vi "PCO Edge_Cam.vi"(0 "Operation":T2(ring), 1 "Camera-specific in":variant, 5 "Exposure time (s)":dbl, 7 "Save path":path, 9 "Capture mode":enum16{"Single frame", "Sequence"}(ring), 12 "Image in":variant, 14 "Frames in sequence":u32=1 min=1) -> (3 "Camera-specific out":variant, 4 "Status":T1)   [LabVIEW 2015]
uses:
  <vilib>/vision/Image Controls.llb/IMAQ Image.ctl
panel:
  in  "Capture button":refnum<vi>
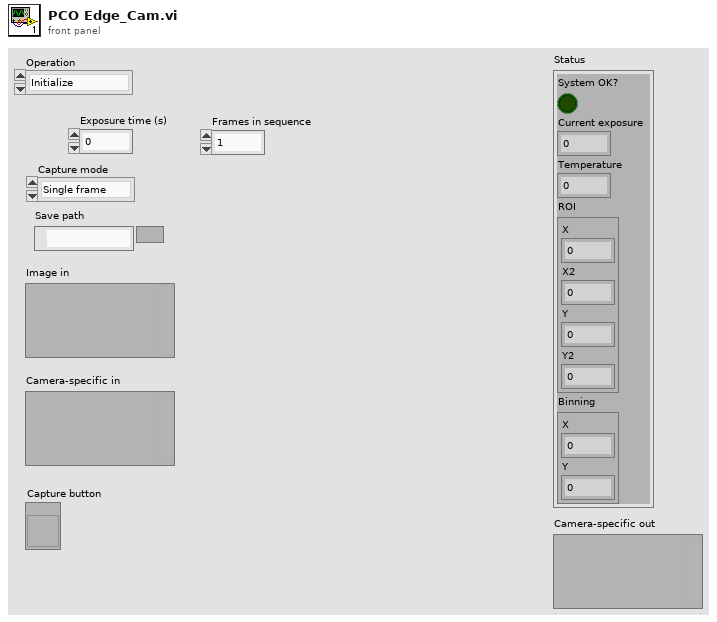
[diagram p1: front panel]
types:
  T1 = cluster{"System OK?":bool, "Current exposure":dbl, "Temperature":dbl, "ROI":cluster{"X":u32, "X2":u32, "Y":u32, "Y2":u32}, "Binning":cluster{"X":u32, "Y":u32}}
  T2 = enum16{"Initialize", "Shut down", "Set capture mode", "Set exposure", "Trigger and read", "Get status", "Other settings"}
  T3 = cluster{"Handle":u64, "Buffers":i16[], "Frames in sequence":u32}
  T4 = cluster{"Size":u16, "InterfaceType":u16, "Camera Number":u16, "CameraNumAtInterface":u16, "OpenFlags":u16[], "OpenDWFlags":u32[], "OpenPtrs":u32[]}
  T5 = typedef "IMAQ Image.ctl" = refnum<image>
  T6 = cluster{"New Image":T5, "Image":refnum<vi>, "FPS target":dbl}
  T7 = enum16{"big-endian, network order", "native, host order", "little-endian"}
  T8 = enum16{"open", "replace", "create", "open or create", "replace or create", "replace or create with confirmation"}
  T9 = cluster{"SSize":u16, "CamType":u16, "CamsSubType":u16, "SerialNumber":u32, "HWVersion":u32, "FWVersion ":u32, "InterfaceType":u16, "HardwareVersions":cluster{"Board":u16, cluster{"string":string, "BatchNumber":u16, "MinorRevision":u8, "MajorRevision":u8, "Variant":u16}[]}, "FirmwareVersions":cluster{"DeviceNum":u16, cluster{"string":string, "MinorRevision":u8, "MajorRevision":u8, "Variant":u16}[]}}
  T10 = cluster{"Size":u16, "SensorTypeDESC":u16, "SensorSubtypeDESC":u16, "MaxHorizontalResStdDESC":u16, "MaxVerticalResStdDESC":u16, "MaxHorizontalResExtDESC":u16, "MaxVerticalResExtDESC":u16, "DynResDESC":u16, "MaxBinHorzDESC":u16, "BinHorzStepDESC":bool, "MaxBinVertDESC":u16, "BinVertStepDESC":bool, "ROIHorzStepDESC":u16, "ROIVertStepDESC":u16, "NumADCDESC":u16, "IRDESC":bool, "MinDelayDESC":u32, "MaxDelayDESC":u32, "MinDelayStepDESC":u32, "MinExpoDESC":u32, "MaxExpoDESC":u32, "MinExpoStepDESC":u32, "MinDelayIRDESC":u32, "MaxDelayIRDESC":u32, "MinExpoIRDESC":u32, "MaxExpoIRDESC":u32, "TimeTableDESC":bool, "DoubleImageDESC":bool, "MinCoolSetDESC":i16, "MaxCoolSetDESC":i16, "MDefaultCoolSetDESC":i16, "PowerDownModeDESC":bool, "OffsetRegDESC":bool, "ColorPattern":cluster{"UpperLeftColor":u8, "UpperRightColor":u8, "LowerLeftColor":u8, "LowerRightColor":u8}, "PatternTypeDESC":bool, "PixelRates":u32[], "CoversionFactors":u16[], "Reserved":u32[], "GeneralCapabilities":u32, "GeneralCapabilities 2":u32, "Min Size Hor":u16, "Min Size Vert":u16, "Ext Synch Freq":u32[], "Cooling Setpoints":i16[], "Soft ROI Hor Step":u16, "Soft ROI Vert Step":u16}
  T11 = cluster{"File refnum":refnum<file>, "Image File Directory":cluster{cluster{"Field":u16, "Type":u16, "Count":u32, "Value / Offset":u32, "Add IFD Offset?":bool}[], cluster{"Data":u32[], "Add offset?":bool}[]}, "Big endian?":bool, "IFD Offset Size":u32}
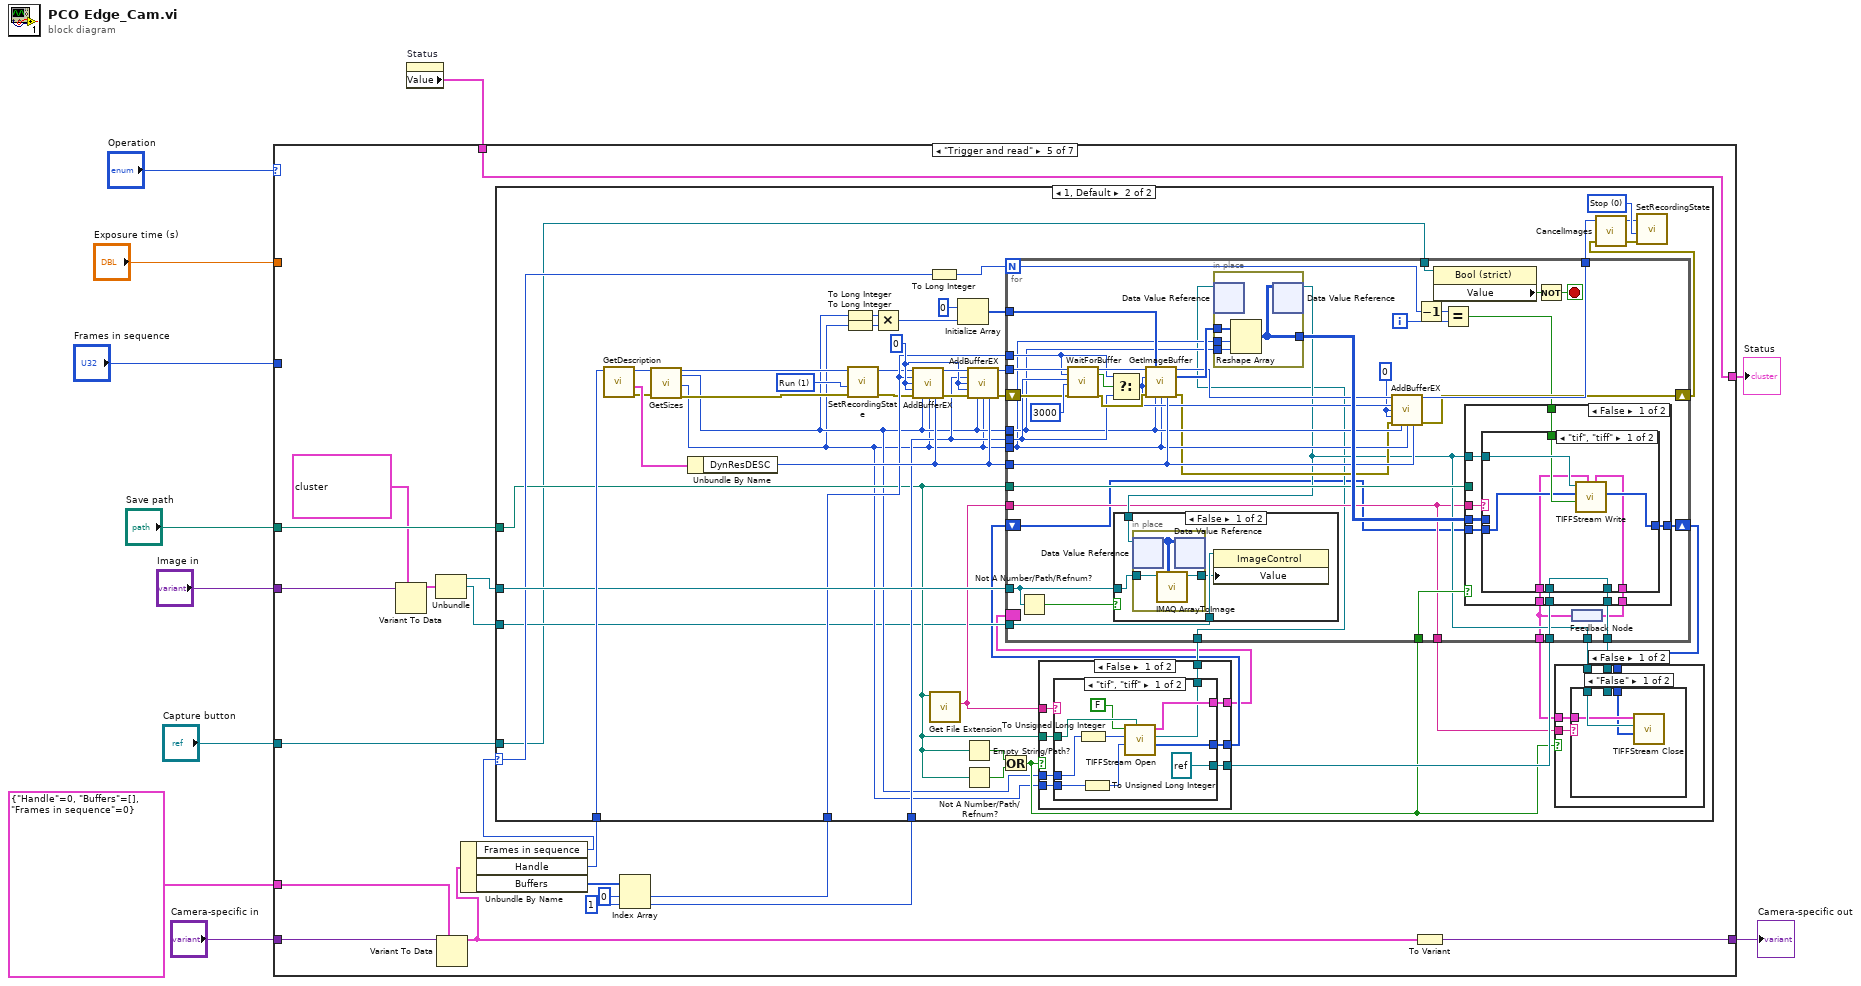
[diagram p0: block diagram]
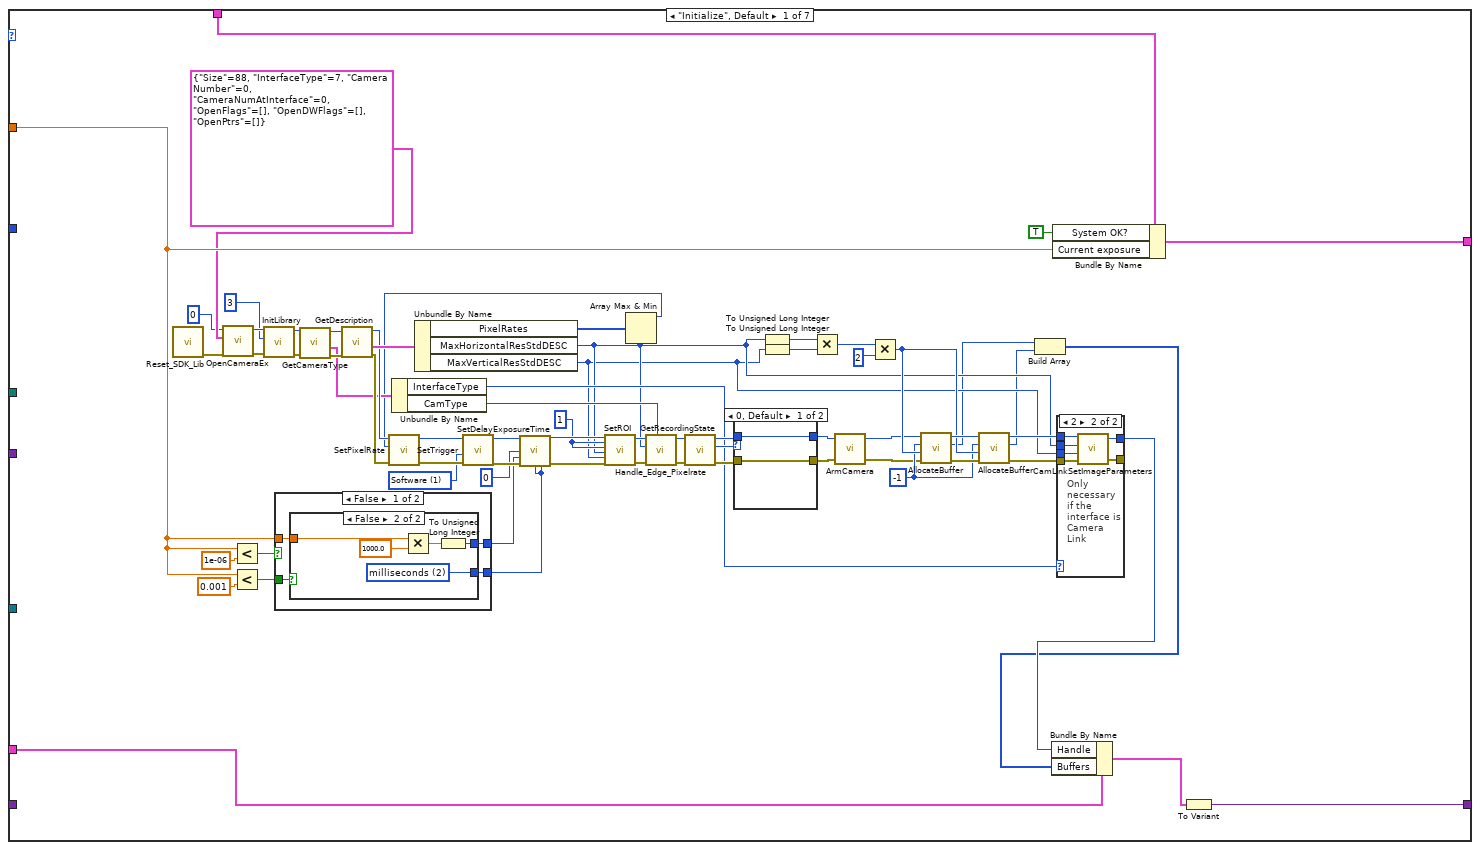
[diagram p2: hidden frame]
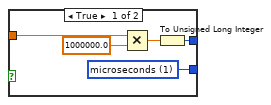
[diagram p3: hidden frame]
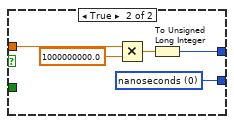
[diagram p4: hidden frame]
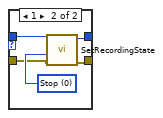
[diagram p6: hidden frame]
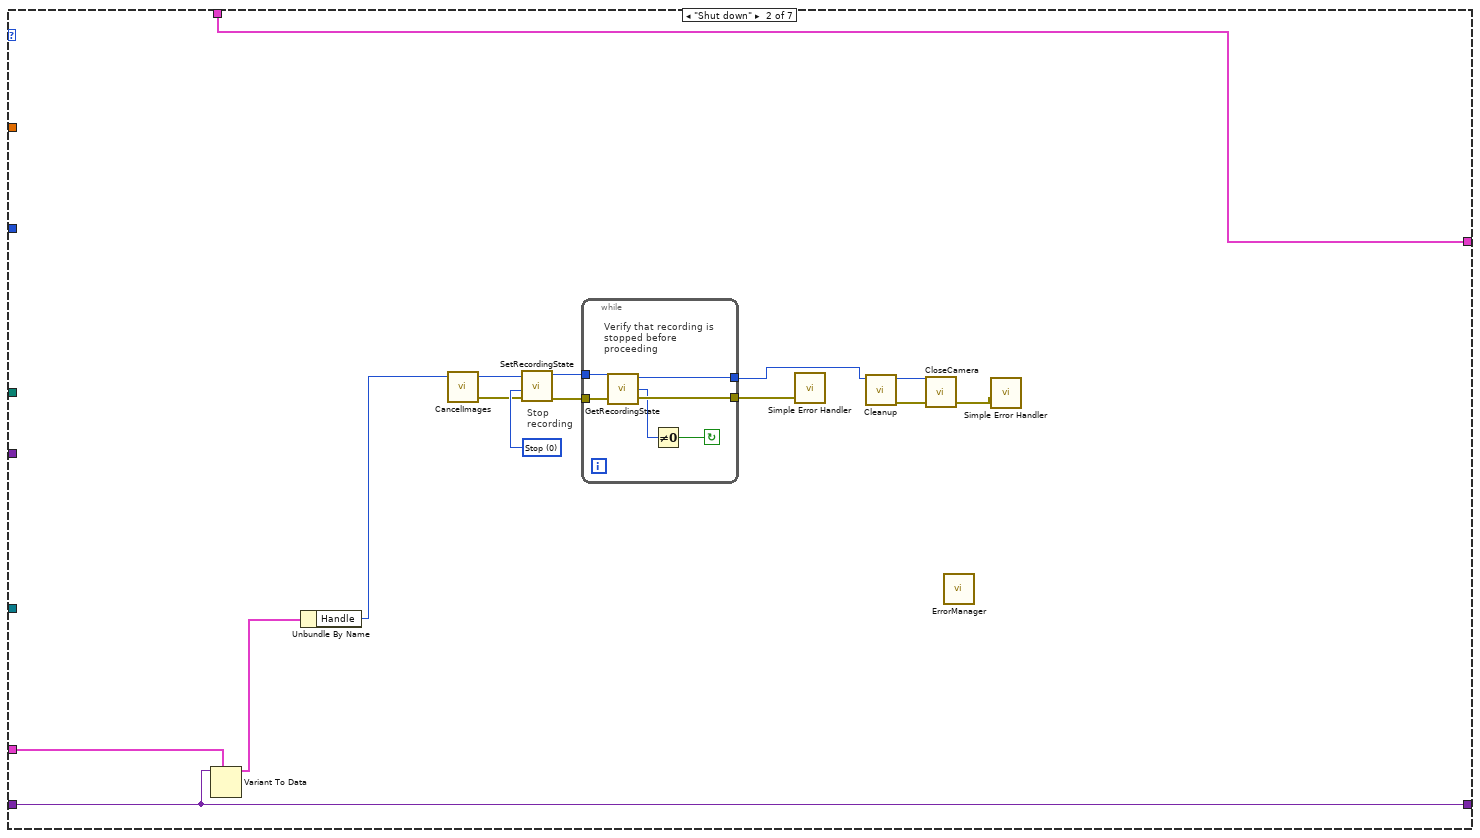
[diagram p7: hidden frame]
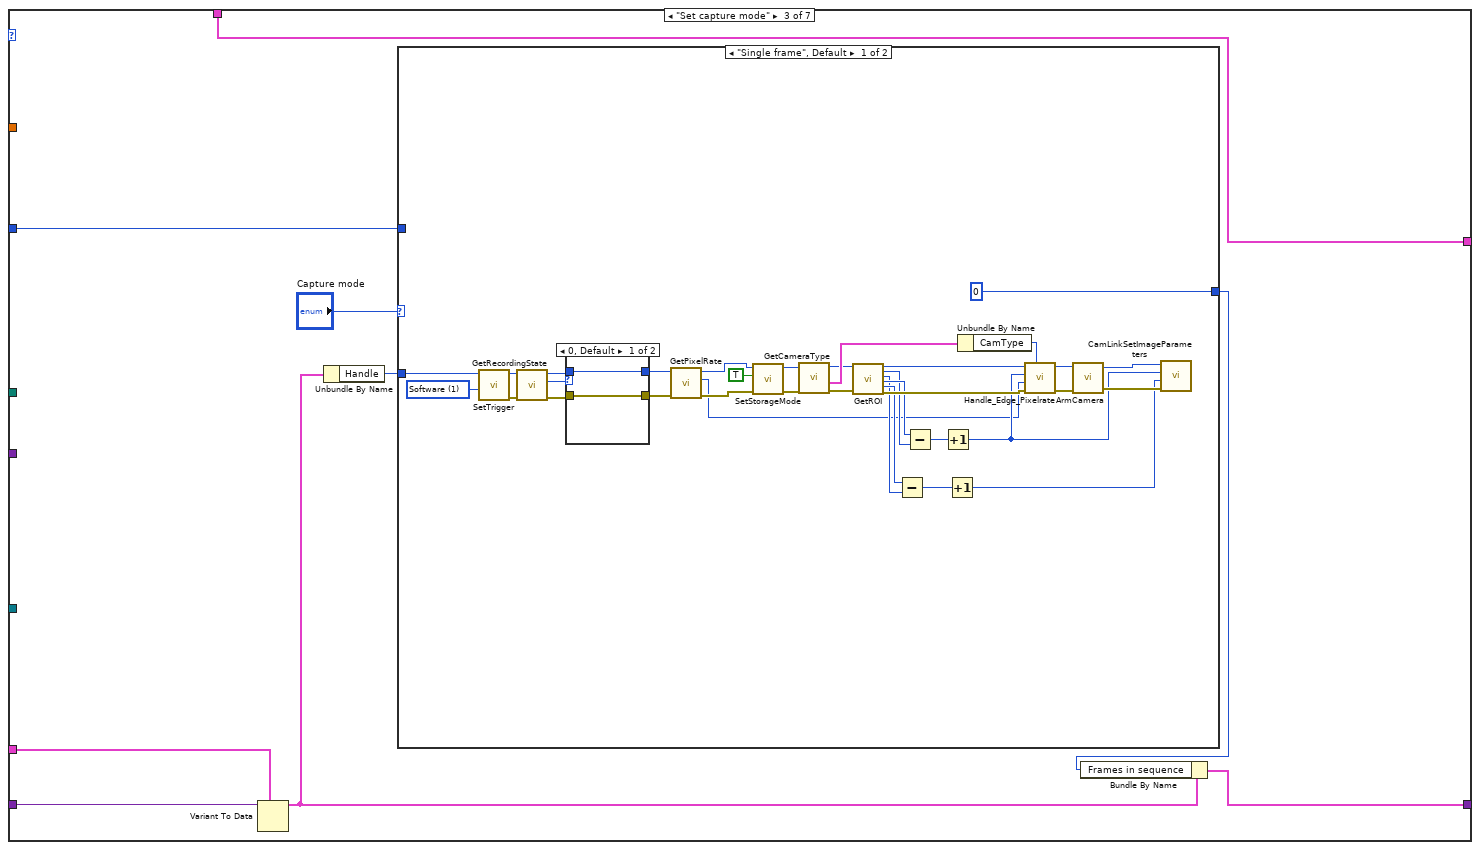
[diagram p8: hidden frame]
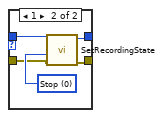
[diagram p9: hidden frame]
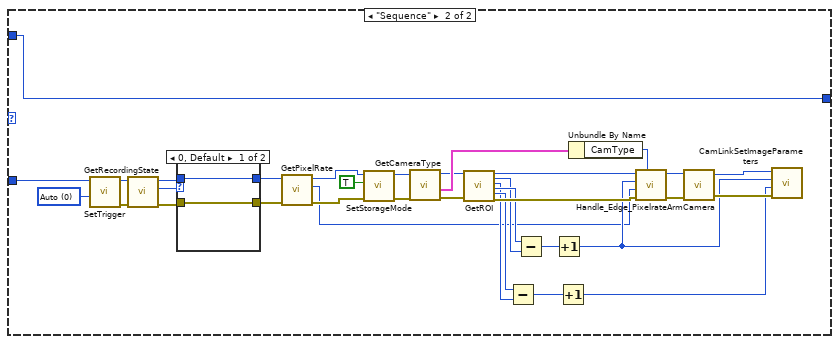
[diagram p10: hidden frame]
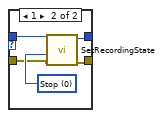
[diagram p11: hidden frame]
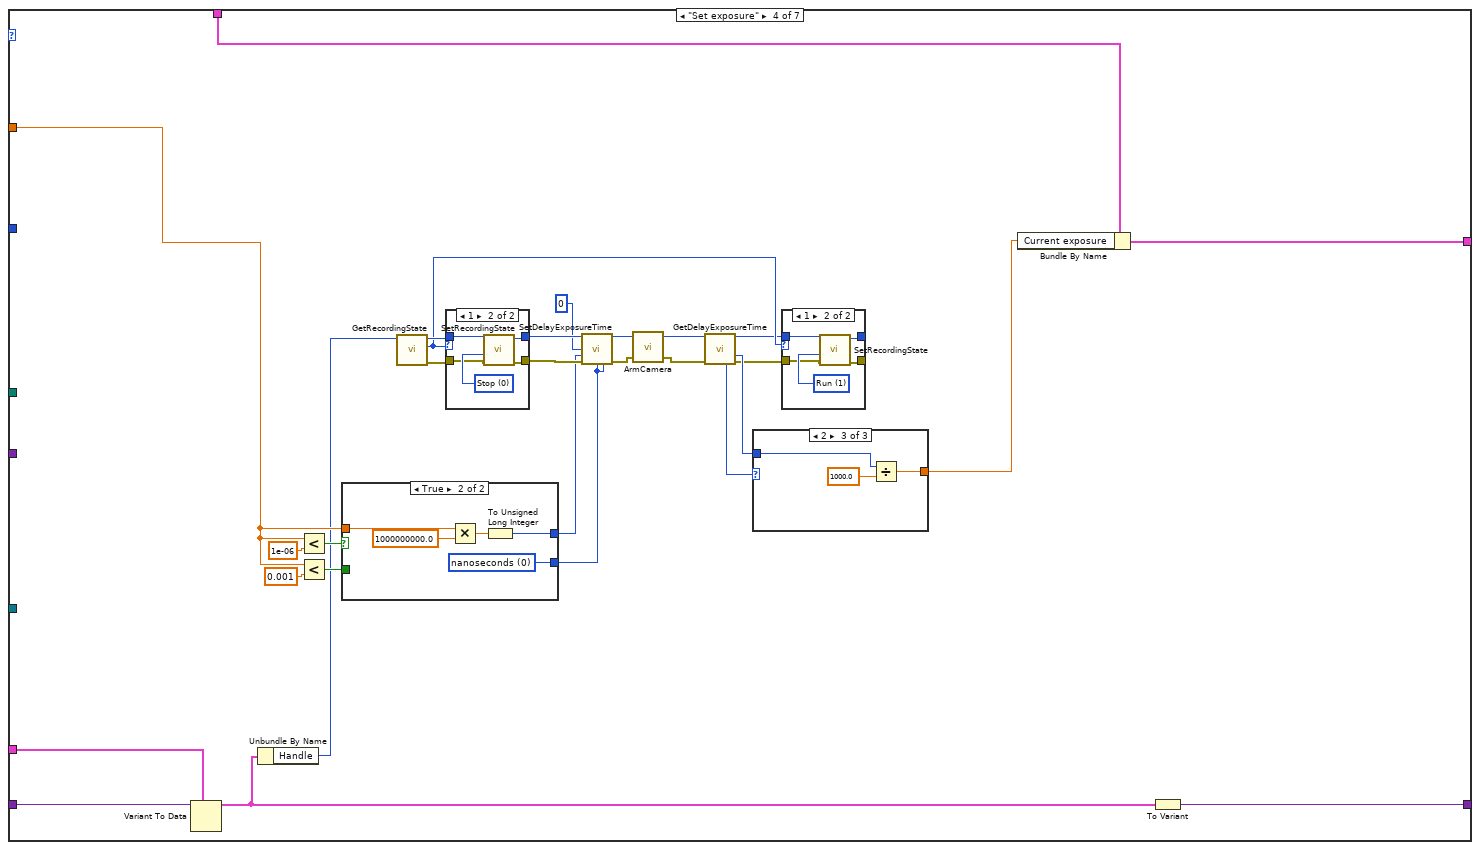
[diagram p12: hidden frame]
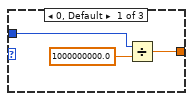
[diagram p14: hidden frame]
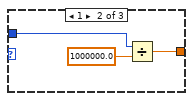
[diagram p15: hidden frame]
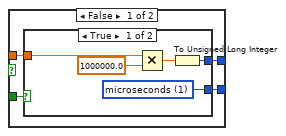
[diagram p16: hidden frame]
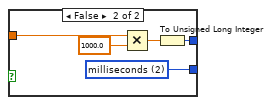
[diagram p17: hidden frame]
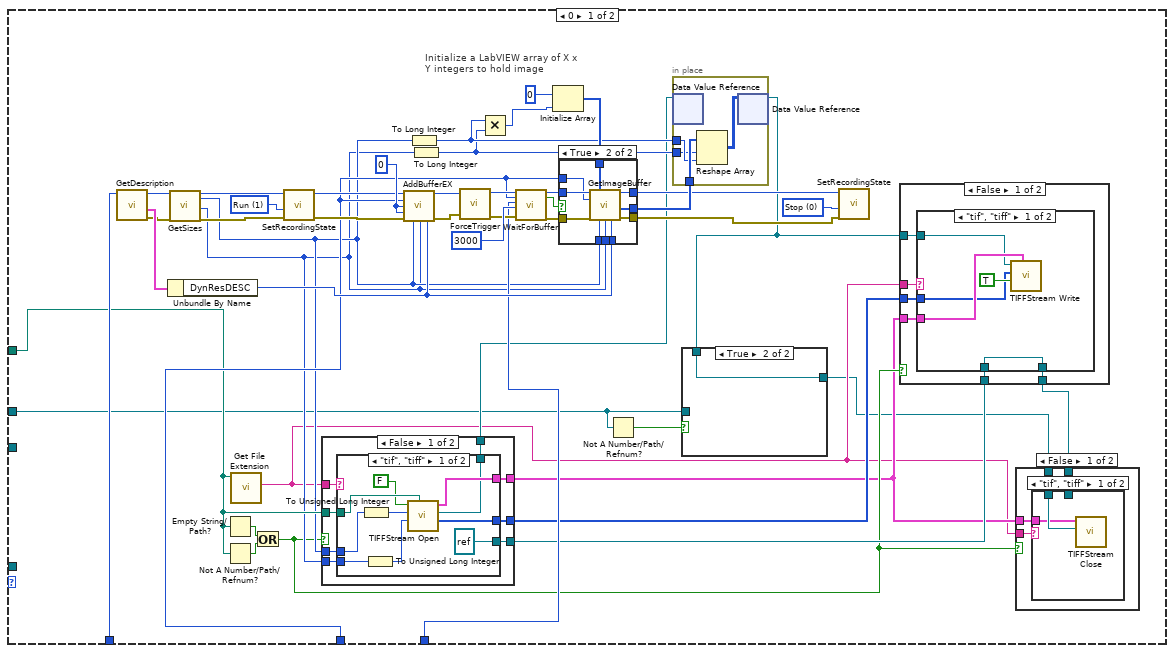
[diagram p19: hidden frame]
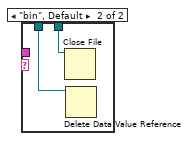
[diagram p20: hidden frame]
diagram:
  n1 = property on="Status" class="Clust (strict)"() -> ("Value"=w9:T1)  [unwired: 2 in, 2 out]
  n2 = case shown="\"Trigger and read\"" "Operation" {
    tunnel: "Exposure time (s)" -> [w27 _ _ w241 _ _ _]
    tunnel: w9 -> [w78 w127 w142 w253 w314 w631 w640]
    tunnel: [w77 w127 w142 w252 w314 w630 w640] -> w8
    tunnel: "Save path" -> [_ _ _ _ w306 _ _]
    tunnel: "Image in" -> [_ _ _ _ w299 _ _]
    tunnel: "Camera-specific in" -> [_ w115 w136 w229 w305 w625 w639]
    tunnel: [w16 w115 w139 w225 w302 w625 w633] -> w3
    tunnel: "Frames in sequence" -> [_ _ w140 _ _ _ _]
    tunnel: T3 {"Handle"=0, "Buffers"=[], "Frames in sequence"=0} -> [w14 w114 w137 w227 w304 _ w635]
    tunnel: "Capture button" -> [_ _ _ _ w296 _ _]
    frame "Initialize", Default {
      w23 = u16 1 ("ROIX0")
      w32 = u16 1 items=["Auto", "Software", "External sequence start ", "External exposure control"] ("TriggerMode")
      w56 = i16 -1
      n3 = call <userlib>:"Reset_SDK_Lib.vi"() -> ("ErrorOut"=w68:errorcluster)  [unwired: 11 in]
      n4 = call <userlib>:"OpenCameraEx.vi"("error in (no error)"=w68, "OpenStructureIn"=T4 {"Size"=88, "InterfaceType"=7, "Camera Number"=0, "CameraNumAtInterface"=0, "OpenFlags"=[], "OpenDWFlags"=[], "OpenPtrs"=[]}, "ph"=u64 0) -> ("error out"=w72:errorcluster, "hout"=w73:u64)  [unwired: 1 in, 2 out]
      n5 = Less?(x=w27, y=1e-06) -> (x < y?=w29:bool)
      n6 = Less?(x=w27, y=0.001) -> (x < y?=w28:bool)
      n7 = call <userlib>:"InitLibrary.vi"("error in (no error)"=w72, "InterfaceType"=u32 3, "ph"=w73) -> ("error out"=w71:errorcluster, "hout"=w70:u64)  [unwired: 7 in]
      n8 = case shown="False" w29 {
        tunnel: [w80 w97] -> w25
        tunnel: w28 -> [w82 _]
        tunnel: w27 -> [w81 w96]
        tunnel: [w79 w93] -> w26
        frame False {
          n9 = case shown="False" w82 {
            tunnel: w81 -> [w84 w89]
            tunnel: [w87 w92] -> w80
            tunnel: [w83 w88] -> w79
            frame True {
              w87 = u16 1 items=["nanoseconds", "microseconds", "milliseconds"] ("ExposureTimeBase")
              n10 = Multiply(x=w84, y=1000000.0) -> (x*y=w85:dbl)
              n11 = To Unsigned Long Integer(number=w85) -> (unsigned 32bit integer=w83:u32)
            }
            frame False {
              w92 = u16 2 items=["nanoseconds", "microseconds", "milliseconds"] ("ExposureTimeBase")
              n12 = Multiply(x=w89, y=1000.0) -> (x*y=w90:dbl)
              n13 = To Unsigned Long Integer(number=w90) -> (unsigned 32bit integer=w88:u32)
            }
          }
        }
        frame True {
          w97 = u16 0 items=["nanoseconds", "microseconds", "milliseconds"] ("ExposureTimeBase")
          n14 = Multiply(x=w96, y=1000000000.0) -> (x*y=w94:dbl)
          n15 = To Unsigned Long Integer(number=w94) -> (unsigned 32bit integer=w93:u32)
        }
      }
      n16 = call <userlib>:"GetCameraType.vi"("ph"=w70, "error in (no error)"=w71) -> ("hout"=w75:u64, "CameraType"=w37:T9, "error out"=w74:errorcluster)  [unwired: 1 in, 1 out]
      n17 = call <userlib>:"GetDescription.vi"("ErrorIn"=w74, "ph"=w75) -> ("ErrorOut"=w47:errorcluster, "Description"=w63:T10, "hout"=w46:u64)  [unwired: 2 in, 1 out]
      n18 = Unbundle By Name(w37) -> ("InterfaceType"=w36:u16, "CamType"=w35:u16)
      n19 = Unbundle By Name(w63) -> ("PixelRates"=w34:u32[], "MaxHorizontalResStdDESC"=w22:u16, "MaxVerticalResStdDESC"=w21:u16)
      n20 = Array Max & Min(array=w34) -> (max value=w33:u32)  [unwired: 3 out]
      n21 = call <userlib>:"SetPixelRate.vi"("error in (no error)"=w47, "PixelRate"=w33, "ph"=w46) -> ("error out"=w54:errorcluster, "hout"=w55:u64)  [unwired: 2 in, 1 out]
      n22 = call <userlib>:"SetTrigger.vi"("error in (no error)"=w54, "TriggerMode"=w32, "ph"=w55) -> ("error out"=w52:errorcluster, "hout"=w53:u64)  [unwired: 2 in, 1 out]
      n23 = call <userlib>:"SetDelayExposureTime.vi"("ph"=w53, "Delay"=u32 0, "Exposure"=w26, "error in (no error)"=w52, "DelayTimeBase"=w25, "ExposureTimeBase"=w25) -> ("hout"=w49:u64, "error out"=w51:errorcluster)  [unwired: 7 in, 1 out]
      n24 = call <userlib>:"SetROI.vi"("ph"=w49, "ROIX0"=w23, "ROIY0"=w23, "ROIX1"=w22, "ROIY1"=w21, "error in (no error)"=w51) -> ("hout"=w48:u64, "error out"=w50:errorcluster)  [unwired: 12 in]
      n25 = call <userlib>:"Handle_Edge_Pixelrate.vi"("Cameratype"=w35, "error in (no error)"=w50, "X-Resolution"=w22, "ph"=w48) -> ("error out"=w44:errorcluster, "hout"=w45:u64)  [unwired: 6 in]
      n26 = call <userlib>:"GetRecordingState.vi"("ErrorIn"=w44, "ph"=w45) -> ("ErrorOut"=w60:errorcluster, "Error"=w58:i32, "hout"=w61:u64)  [unwired: 2 in, 1 out]
      n27 = case shown="0, Default" w58 {
        tunnel: w61 -> [w107 w111]
        tunnel: w60 -> [w106 w110]
        tunnel: [w107 w109] -> w43
        tunnel: [w106 w108] -> w41
        frame 0, Default {
        }
        frame 1 {
          w112 = u16 0 items=["Stop", "Run"] ("RecordingState")
          n28 = call <userlib>:"SetRecordingState.vi"("ErrorIn"=w110, "RecordingState"=w112, "ph"=w111) -> ("ErrorOut"=w108:errorcluster, "hout"=w109:u64)  [unwired: 2 in, 1 out]
        }
      }
      n29 = To Unsigned Long Integer(number=w22) -> (unsigned 32bit integer=w65:u32)
      n30 = To Unsigned Long Integer(number=w21) -> (unsigned 32bit integer=w64:u32)
      n31 = Multiply(x=w65, y=w64) -> (x*y=w66:u32)
      n32 = call <userlib>:"ArmCamera.vi"("error in (no error)"=w41, "ph"=w43) -> ("error out"=w40:errorcluster, "hout"=w42:u64)  [unwired: 1 in, 1 out]
      n33 = Multiply(x=w66, y=u32 2) -> (x*y=w57:u32)
      n34 = call <userlib>:"AllocateBuffer.vi"("error in (no error)"=w40, "Size"=w57, "BufNr"=w56, "ph"=w42) -> ("error out"=w62:errorcluster, "BufNrOut"=w20:i16, "hout"=w59:u64)  [unwired: 2 in, 3 out]
      n35 = call <userlib>:"AllocateBuffer.vi"("error in (no error)"=w62, "Size"=w57, "BufNr"=w56, "ph"=w59) -> ("error out"=w38:errorcluster, "BufNrOut"=w19:i16, "hout"=w39:u64)  [unwired: 2 in, 3 out]
      n36 = Build Array(w20, w19) -> (w17:i16[])
      n37 = Bundle By Name(cluster=w78, "System OK?"=TRUE, "Current exposure"=w27) -> (w77:T1)
      n38 = case shown="2" w36 {
        tunnel: w38 -> [w98 w105]
        tunnel: [w98 w104] -> _
        tunnel: w39 -> [w99 w103]
        tunnel: [w99 w102] -> w18
        tunnel: w21 -> [_ w101]
        tunnel: w22 -> [_ w100]
        frame 0, Default {
        }
        frame 2 {
          # "Only necessary if the interface is Camera Link"
          n39 = call <userlib>:"CamLinkSetImageParameters.vi"("error in (no error)"=w105, "YRes"=w101, "XRes"=w100, "ph"=w103) -> ("error out"=w104:errorcluster, "hout"=w102:u64)  [unwired: 1 out]
        }
      }
      n40 = Bundle By Name(cluster=w14, "Handle"=w18, "Buffers"=w17) -> (w15:T3)
      n41 = To Variant(anything=w15) -> (Variant=w16:variant)
    }
    frame "Shut down" {
      w126 = u16 0 items=["Stop", "Run"] ("RecordingState")
      # "Stop recording"
      n42 = Variant To Data(type=w114, Variant=w115) -> (data=w113:T3)  [unwired: 1 in, 1 out]
      n43 = Unbundle By Name(w113) -> ("Handle"=w116:u64)
      n44 = call <userlib>:"CancelImages.vi"("ph"=w116) -> ("error out"=w123:errorcluster, "hout"=w122:u64)  [unwired: 2 in, 1 out]
      n45 = call <userlib>:"SetRecordingState.vi"("ErrorIn"=w123, "RecordingState"=w126, "ph"=w122) -> ("ErrorOut"=w124:errorcluster, "hout"=w125:u64)  [unwired: 2 in, 1 out]
      n46 = while {
        tunnel: [w131] -> w121
        tunnel: w124 -> [w132]
        tunnel: w125 -> [w133]
        tunnel: [w128] -> w117
        stop <- w129 continue-if-true
        # "Verify that recording is stopped before proceeding"
        n47 = call <userlib>:"GetRecordingState.vi"("ErrorIn"=w132, "ph"=w133) -> ("ErrorOut"=w131:errorcluster, "RecordingState"=w130:u16, "hout"=w128:u64)  [unwired: 2 in, 1 out]
        n48 = Not Equal To 0?(x=w130) -> (x != 0?=w129:bool)
      }
      n49 = call <vilib>:"Simple Error Handler.vi"("error in (no error)"=w121) -> ()  [unwired: 4 in, 5 out]
      n50 = call <userlib>:"Cleanup.vi"("ph"=w117) -> ("error out"=w118:errorcluster, "hout"=w119:u64)  [unwired: 9 in]
      n51 = call <userlib>:"CloseCamera.vi"("ErrorIn"=w118, "Handle in"=w119) -> ("ErrorOut"=w120:errorcluster)  [unwired: 1 in, 2 out]
      n52 = call <userlib>:"ErrorManager.vi"() -> ()  [unwired: 5 in, 1 out]
      n53 = call <vilib>:"Simple Error Handler.vi"("error in (no error)"=w120) -> ()  [unwired: 4 in, 5 out]
    }
    frame "Set capture mode" {
      n54 = Variant To Data(type=w137, Variant=w136) -> (data=w135:T3)  [unwired: 1 in, 1 out]
      n55 = Unbundle By Name(w135) -> ("Handle"=w138:u64)
      n56 = case shown="\"Single frame\", Default" "Capture mode" {
        tunnel: w140 -> [_ w184]
        tunnel: [u32 0 ("Frames in sequence") w184] -> w134
        tunnel: w138 -> [w174 w216]
        frame "Single frame", Default {
          w175 = u16 1 items=["Auto", "Software", "External sequence start ", "External exposure control"] ("TriggerMode")
          n57 = call <userlib>:"SetTrigger.vi"("TriggerMode"=w175, "ph"=w174) -> ("error out"=w169:errorcluster, "hout"=w170:u64)  [unwired: 3 in, 1 out]
          n58 = call <userlib>:"GetRecordingState.vi"("ErrorIn"=w169, "ph"=w170) -> ("ErrorOut"=w172:errorcluster, "Error"=w171:i32, "hout"=w173:u64)  [unwired: 2 in, 1 out]
          n59 = case shown="0, Default" w171 {
            tunnel: w173 -> [w178 w182]
            tunnel: w172 -> [w177 w181]
            tunnel: [w178 w180] -> w146
            tunnel: [w177 w179] -> w145
            frame 0, Default {
            }
            frame 1 {
              w183 = u16 0 items=["Stop", "Run"] ("RecordingState")
              n60 = call <userlib>:"SetRecordingState.vi"("ErrorIn"=w181, "RecordingState"=w183, "ph"=w182) -> ("ErrorOut"=w179:errorcluster, "hout"=w180:u64)  [unwired: 2 in, 1 out]
            }
          }
          n61 = call <userlib>:"GetPixelRate.vi"("error in (no error)"=w145, "ph"=w146) -> ("error out"=w144:errorcluster, "PixelRate"=w143:u32, "hout"=w147:u64)  [unwired: 2 in, 1 out]
          n62 = call <userlib>:"SetStorageMode.vi"("error in (no error)"=w144, "StorageMode"=TRUE, "ph"=w147) -> ("error out"=w161:errorcluster, "hout"=w162:u64)  [unwired: 2 in, 1 out]
          n63 = call <userlib>:"GetCameraType.vi"("ph"=w162, "error in (no error)"=w161) -> ("hout"=w157:u64, "CameraType"=w168:T9, "error out"=w159:errorcluster)  [unwired: 1 in, 1 out]
          n64 = call <userlib>:"GetROI.vi"("ph"=w157, "error in (no error)"=w159) -> ("hout"=w156:u64, "ROIX0"=w154:u16, "ROIY0"=w152:u16, "ROIX1"=w155:u16, "ROIY1"=w153:u16, "error out"=w158:errorcluster)  [unwired: 12 in]
          n65 = Subtract(x=w153, y=w152) -> (x-y=w150:u16)
          n66 = Subtract(x=w155, y=w154) -> (x-y=w151:u16)
          n67 = Increment(x=w151) -> (x+1=w149:u16)
          n68 = Increment(x=w150) -> (x+1=w148:u16)
          n69 = Unbundle By Name(w168) -> ("CamType"=w167:u16)
          n70 = call <userlib>:"Handle_Edge_Pixelrate.vi"("Cameratype"=w167, "error in (no error)"=w158, "PixelRate"=w143, "X-Resolution"=w149, "ph"=w156) -> ("error out"=w163:errorcluster, "hout"=w164:u64)  [unwired: 5 in]
          n71 = call <userlib>:"ArmCamera.vi"("error in (no error)"=w163, "ph"=w164) -> ("error out"=w166:errorcluster, "hout"=w165:u64)  [unwired: 1 in, 1 out]
          n72 = call <userlib>:"CamLinkSetImageParameters.vi"("error in (no error)"=w166, "YRes"=w148, "XRes"=w149, "ph"=w165) -> ()  [unwired: 3 out]
        }
        frame "Sequence" {
          w217 = u16 0 items=["Auto", "Software", "External sequence start ", "External exposure control"] ("TriggerMode")
          n73 = call <userlib>:"SetTrigger.vi"("TriggerMode"=w217, "ph"=w216) -> ("error out"=w211:errorcluster, "hout"=w212:u64)  [unwired: 3 in, 1 out]
          n74 = call <userlib>:"GetRecordingState.vi"("ErrorIn"=w211, "ph"=w212) -> ("ErrorOut"=w214:errorcluster, "Error"=w213:i32, "hout"=w215:u64)  [unwired: 2 in, 1 out]
          n75 = case shown="0, Default" w213 {
            tunnel: w215 -> [w219 w223]
            tunnel: w214 -> [w218 w222]
            tunnel: [w219 w221] -> w188
            tunnel: [w218 w220] -> w187
            frame 0, Default {
            }
            frame 1 {
              w224 = u16 0 items=["Stop", "Run"] ("RecordingState")
              n76 = call <userlib>:"SetRecordingState.vi"("ErrorIn"=w222, "RecordingState"=w224, "ph"=w223) -> ("ErrorOut"=w220:errorcluster, "hout"=w221:u64)  [unwired: 2 in, 1 out]
            }
          }
          n77 = call <userlib>:"GetPixelRate.vi"("error in (no error)"=w187, "ph"=w188) -> ("error out"=w186:errorcluster, "PixelRate"=w185:u32, "hout"=w189:u64)  [unwired: 2 in, 1 out]
          n78 = call <userlib>:"SetStorageMode.vi"("error in (no error)"=w186, "StorageMode"=TRUE, "ph"=w189) -> ("error out"=w203:errorcluster, "hout"=w204:u64)  [unwired: 2 in, 1 out]
          n79 = call <userlib>:"GetCameraType.vi"("ph"=w204, "error in (no error)"=w203) -> ("hout"=w199:u64, "CameraType"=w210:T9, "error out"=w201:errorcluster)  [unwired: 1 in, 1 out]
          n80 = call <userlib>:"GetROI.vi"("ph"=w199, "error in (no error)"=w201) -> ("hout"=w198:u64, "ROIX0"=w196:u16, "ROIY0"=w194:u16, "ROIX1"=w197:u16, "ROIY1"=w195:u16, "error out"=w200:errorcluster)  [unwired: 12 in]
          n81 = Subtract(x=w195, y=w194) -> (x-y=w192:u16)
          n82 = Subtract(x=w197, y=w196) -> (x-y=w193:u16)
          n83 = Increment(x=w193) -> (x+1=w191:u16)
          n84 = Increment(x=w192) -> (x+1=w190:u16)
          n85 = Unbundle By Name(w210) -> ("CamType"=w209:u16)
          n86 = call <userlib>:"Handle_Edge_Pixelrate.vi"("Cameratype"=w209, "error in (no error)"=w200, "PixelRate"=w185, "X-Resolution"=w191, "ph"=w198) -> ("error out"=w205:errorcluster, "hout"=w206:u64)  [unwired: 5 in]
          n87 = call <userlib>:"ArmCamera.vi"("error in (no error)"=w205, "ph"=w206) -> ("error out"=w208:errorcluster, "hout"=w207:u64)  [unwired: 1 in, 1 out]
          n88 = call <userlib>:"CamLinkSetImageParameters.vi"("error in (no error)"=w208, "YRes"=w190, "XRes"=w191, "ph"=w207) -> ()  [unwired: 3 out]
        }
      }
      n89 = Bundle By Name(cluster=w135, "Frames in sequence"=w134) -> (w139:T3)
    }
    frame "Set exposure" {
      n90 = Variant To Data(type=w227, Variant=w229) -> (data=w226:T3)  [unwired: 1 in, 1 out]
      n91 = Unbundle By Name(w226) -> ("Handle"=w228:u64)
      n92 = Less?(x=w241, y=1e-06) -> (x < y?=w243:bool)
      n93 = Less?(x=w241, y=0.001) -> (x < y?=w242:bool)
      n94 = case shown="True" w243 {
        tunnel: [w271 w288] -> w238
        tunnel: w242 -> [w273 _]
        tunnel: w241 -> [w272 w287]
        tunnel: [w270 w284] -> w239
        frame False {
          n95 = case shown="True" w273 {
            tunnel: w272 -> [w275 w280]
            tunnel: [w278 w283] -> w271
            tunnel: [w274 w279] -> w270
            frame True {
              w278 = u16 1 items=["nanoseconds", "microseconds", "milliseconds"] ("ExposureTimeBase")
              n96 = Multiply(x=w275, y=1000000.0) -> (x*y=w276:dbl)
              n97 = To Unsigned Long Integer(number=w276) -> (unsigned 32bit integer=w274:u32)
            }
            frame False {
              w283 = u16 2 items=["nanoseconds", "microseconds", "milliseconds"] ("ExposureTimeBase")
              n98 = Multiply(x=w280, y=1000.0) -> (x*y=w281:dbl)
              n99 = To Unsigned Long Integer(number=w281) -> (unsigned 32bit integer=w279:u32)
            }
          }
        }
        frame True {
          w288 = u16 0 items=["nanoseconds", "microseconds", "milliseconds"] ("ExposureTimeBase")
          n100 = Multiply(x=w287, y=1000000000.0) -> (x*y=w285:dbl)
          n101 = To Unsigned Long Integer(number=w285) -> (unsigned 32bit integer=w284:u32)
        }
      }
      n102 = call <userlib>:"GetRecordingState.vi"("ph"=w228) -> ("ErrorOut"=w250:errorcluster, "Error"=w233:i32, "hout"=w251:u64)  [unwired: 3 in, 1 out]
      n103 = case shown="1" w233 {
        tunnel: w251 -> [w290 w294]
        tunnel: w250 -> [w289 w293]
        tunnel: [w290 w292] -> w249
        tunnel: [w289 w291] -> w246
        frame 0, Default {
        }
        frame 1 {
          w295 = u16 0 items=["Stop", "Run"] ("RecordingState")
          n104 = call <userlib>:"SetRecordingState.vi"("ErrorIn"=w293, "RecordingState"=w295, "ph"=w294) -> ("ErrorOut"=w291:errorcluster, "hout"=w292:u64)  [unwired: 2 in, 1 out]
        }
      }
      n105 = call <userlib>:"SetDelayExposureTime.vi"("ph"=w249, "Delay"=u32 0, "Exposure"=w239, "error in (no error)"=w246, "DelayTimeBase"=w238, "ExposureTimeBase"=w238) -> ("hout"=w248:u64, "error out"=w247:errorcluster)  [unwired: 7 in, 1 out]
      n106 = call <userlib>:"ArmCamera.vi"("error in (no error)"=w247, "ph"=w248) -> ("error out"=w236:errorcluster, "hout"=w237:u64)  [unwired: 1 in, 1 out]
      n107 = call <userlib>:"GetDelayExposureTime.vi"("ph"=w237, "error in (no error)"=w236) -> ("hout"=w232:u64, "Exposure"=w234:u32, "ExposureTimeBase"=w235:u16, "error out"=w231:errorcluster)  [unwired: 7 in, 3 out]
      n108 = case shown="2" w235 {
        tunnel: w234 -> [w263 w266 w269]
        tunnel: [w261 w264 w267] -> w230
        frame 0, Default {
          n109 = Divide(x=w263, y=1000000000.0) -> (x/y=w261:dbl)
        }
        frame 1 {
          n110 = Divide(x=w266, y=1000000.0) -> (x/y=w264:dbl)
        }
        frame 2 {
          n111 = Divide(x=w269, y=1000.0) -> (x/y=w267:dbl)
        }
      }
      n112 = case shown="1" w233 {
        tunnel: w232 -> [w255 w259]
        tunnel: w231 -> [w254 w258]
        tunnel: [w255 w257] -> _
        tunnel: [w254 w256] -> _
        frame 0, Default {
        }
        frame 1 {
          w260 = u16 1 items=["Stop", "Run"] ("RecordingState")
          n113 = call <userlib>:"SetRecordingState.vi"("ErrorIn"=w258, "RecordingState"=w260, "ph"=w259) -> ("ErrorOut"=w256:errorcluster, "hout"=w257:u64)  [unwired: 2 in, 1 out]
        }
      }
      n114 = Bundle By Name(cluster=w253, "Current exposure"=w230) -> (w252:T1)
      n115 = To Variant(anything=w226) -> (Variant=w225:variant)
    }
    frame "Trigger and read" {
      n116 = Variant To Data(type=T6 {"New Image"=refnum, "Image"=refnum, "FPS target"=0.0} ("output cluster"), Variant=w299) -> (data=w301:T6)  [unwired: 1 in, 1 out]
      n117 = Unbundle(w301) -> ("New Image"=w298:T5, "Image"=w297:refnum<vi>)  [unwired: 1 out]
      n118 = Variant To Data(type=w304, Variant=w305) -> (data=w303:T3)  [unwired: 1 in, 1 out]
      n119 = Unbundle By Name(w303) -> ("Frames in sequence"=w307:u32, "Handle"=w308:u64, "Buffers"=w313:i16[])
      n120 = Index Array(array=w313, index #1=0 ("index"), index #2=1 ("index")) -> (element #1=w310:i16, element #2=w309:i16)
      n121 = case shown="1, Default" w307 {
        selector: w307 -> [_ w491]
        tunnel: w310 -> [w330 w483]
        tunnel: w309 -> [w329 w485]
        tunnel: w308 -> [w349 w495]
        tunnel: w298 -> [w324 w493]
        tunnel: w306 -> [w328 w462]
        tunnel: w297 -> [_ w454]
        tunnel: w296 -> [_ w451]
        frame 0 {
          w343 = u16 0 items=["Stop", "Run"] ("RecordingState")
          w346 = u16 1 items=["Stop", "Run"] ("RecordingState")
          w356 = u32 0
          # "Initialize a LabVIEW array of X x Y integers to hold image"
          n122 = call <userlib>:"GetDescription.vi"("ph"=w349) -> ("ErrorOut"=w336:errorcluster, "Description"=w348:T10, "hout"=w334:u64)  [unwired: 3 in, 1 out]
          n123 = Unbundle By Name(w348) -> ("DynResDESC"=w347:u16)
          n124 = call <userlib>:"GetSizes.vi"("ph"=w334, "ErrorIn"=w336) -> ("hout"=w333:u64, "XResAct"=w327:u16, "YResAct"=w326:u16, "ErrorOut"=w335:errorcluster)  [unwired: 11 in, 3 out]
          n125 = Empty String/Path?(string/path=w328) -> (empty?=w331:bool)
          n126 = Not A Number/Path/Refnum?(number/path/refnum=w328) -> (NaN/Path/Refnum?=w332:bool)
          n127 = call <vilib>:"Get File Extension.vi"("file"=w328) -> ("lowercase file extension"=w317:string)  [unwired: 6 in, 4 out]
          n128 = Or(x=w331, y=w332) -> (x .or. y?=w320:bool)
          n129 = call <userlib>:"SetRecordingState.vi"("ErrorIn"=w335, "RecordingState"=w346, "ph"=w333) -> ("ErrorOut"=w344:errorcluster, "hout"=w345:u64)  [unwired: 2 in, 1 out]
          n130 = case shown="False" w320 {
            tunnel: w328 -> [w403 _]
            tunnel: [w402 refnum<file> refnum ("refnum out")] -> w323
            tunnel: w317 -> [w401 _]
            tunnel: [w400 _] -> w318
            tunnel: [w399 w426] -> w325
            tunnel: [w398 _] -> w322
            tunnel: w327 -> [w397 w429]
            tunnel: w326 -> [w396 w430]
            frame False {
              n131 = case shown="\"tif\", \"tiff\"" w401 {
                tunnel: w403 -> [w412 w423]
                tunnel: [refnum<file> refnum ("refnum out") w421] -> w402
                tunnel: [w411 _] -> w400
                tunnel: [w410 w416] -> w399
                tunnel: [w409 _] -> w398
                tunnel: w397 -> [w408 w414]
                tunnel: w396 -> [w407 w415]
                frame "tif", "tiff" {
                  n132 = To Unsigned Long Integer(number=w408) -> (unsigned 32bit integer=w405:u32)
                  n133 = To Unsigned Long Integer(number=w407) -> (unsigned 32bit integer=w406:u32)
                  n134 = call "TIFFStream Open.vi"("File path"=w412, "Height Pixels"=w406, "Width Pixels"=w405, "Big endian?"=FALSE) -> ("Current and next IFD offset"=w409:u32[], "Image data reference"=w410:refnum<data-value>, "File data"=w411:T11)  [unwired: 4 in, 1 out]
                }
                frame "bin", Default {
                  n135 = To Long Integer(number=w415) -> (32bit integer=w417:i32)
                  n136 = To Long Integer(number=w414) -> (32bit integer=w418:i32)
                  n137 = Open/Create/Replace File(file path (use dialog)=w423, operation (0:open)=T8."replace or create") -> (refnum out=w421:refnum<file>)  [unwired: 4 in, 2 out]
                  n138 = Initialize Array(u16 0 ("element"), w417, w418) -> (w419:u16[][])
                  n139 = New Data Value Reference(data value=w419) -> (data value reference=w416:refnum<data-value>)  [unwired: 1 in, 1 out]
                }
              }
            }
            frame True {
              n140 = To Long Integer(number=w430) -> (32bit integer=w424:i32)
              n141 = To Long Integer(number=w429) -> (32bit integer=w425:i32)
              n142 = Initialize Array(u16 0 ("element"), w424, w425) -> (w427:u16[][])
              n143 = New Data Value Reference(data value=w427) -> (data value reference=w426:refnum<data-value>)  [unwired: 1 in, 1 out]
            }
          }
          n144 = call <userlib>:"AddBufferEX.vi"("ph"=w345, "BuffNr"=w330, "1stImage"=w356, "LastImage"=w356, "error in (no error)"=w344, "XRes"=w327, "YRes"=w326, "BitPerPixel"=w347) -> ("hout"=w355:u64, "error out"=w354:errorcluster)  [unwired: 5 in, 1 out]
          n145 = To Long Integer(number=w327) -> (32bit integer=w339:i32)
          n146 = To Long Integer(number=w326) -> (32bit integer=w338:i32)
          n147 = call <userlib>:"ForceTrigger.vi"("ph"=w355, "error in (no error)"=w354) -> ("hout"=w352:u64, "error out"=w353:errorcluster)  [unwired: 1 in, 2 out]
          n148 = Multiply(x=w339, y=w338) -> (x*y=w337:i32)
          n149 = call <userlib>:"WaitForBuffer.vi"("ph"=w352, "sBufNr"=w330, "sBufNr 2"=w329, "timeout"=u32 3000, "error in (no error)"=w353) -> ("hout"=w359:u64, "Buffer_Ready"=w340:bool, "error out"=w358:errorcluster)  [unwired: 10 in, 2 out]
          n150 = Initialize Array(u16 0 ("Element Data"), w337) -> (w350:u16[])
          n151 = case shown="True" w340 {
            tunnel: [w438 w448] -> w360
            tunnel: w359 -> [w436 w447]
            tunnel: w358 -> [w437 w446]
            tunnel: w350 -> [w438 w445]
            tunnel: w347 -> [_ w444]
            tunnel: w327 -> [_ w443]
            tunnel: w326 -> [_ w442]
            tunnel: w330 -> [_ w441]
            tunnel: [w436 w440] -> w342
            tunnel: [w437 w439] -> w341
            frame False {
            }
            frame True {
              n152 = call <userlib>:"GetImageBuffer.vi"("ph"=w447, "BuffIn"=w445, "BuffNr"=w441, "error in (no error)"=w446, "xRes"=w443, "yRes"=w442, "Bitresolution"=w444) -> ("hout"=w440:u64, "BuffOut"=w448:u16[], "error out"=w439:errorcluster)  [unwired: 5 in, 1 out]
            }
          }
          n153 = Not A Number/Path/Refnum?(number/path/refnum=w324) -> (NaN/Path/Refnum?=w321:bool)
          n154 = in-place {
            in-place-border: w360 -> [w435]
            in-place-border: w339 -> [w434]
            in-place-border: w338 -> [w433]
            n155 = in-place-dvr #1(w325) -> ()  [unwired: 2 out]
            n156 = Reshape Array(w435, w433, w434) -> (w432:u16[][])
            n157 = in-place-dvr #1(w432) -> (w316:refnum<data-value>)  [unwired: 1 out]
          }
          n158 = case shown="True" w321 {
            tunnel: w324 -> [w391 _]
            tunnel: w316 -> [w390 w395]
            tunnel: [w389 w395] -> w315
            frame False {
              n159 = in-place {
                in-place-border: w391 -> [w394]
                n160 = in-place-dvr #2(w390) -> (w393:u16[][], w392:errorcluster)
                n161 = call "IMAQ ArrayToImage"("Image Pixels (U16)"=w393, "error in (no error)"=w392, "Image"=w394) -> ()  [unwired: 7 in, 2 out]
                n162 = in-place-dvr #2(w393) -> (w389:refnum<data-value>)  [unwired: 1 out]
              }
            }
            frame True {
            }
          }
          n163 = call <userlib>:"SetRecordingState.vi"("ErrorIn"=w341, "RecordingState"=w343, "ph"=w342) -> ()  [unwired: 2 in, 3 out]
          n164 = case shown="False" w320 {
            tunnel: w322 -> [w374 _]
            tunnel: w323 -> [w373 w388]
            tunnel: [w372 w388] -> w319
            tunnel: w317 -> [w371 _]
            tunnel: w318 -> [w370 _]
            tunnel: w316 -> [w369 _]
            frame False {
              n165 = case shown="\"tif\", \"tiff\"" w371 {
                tunnel: w374 -> [w375 _]
                tunnel: w373 -> [w378 w382]
                tunnel: [w378 w381] -> w372
                tunnel: w370 -> [w379 _]
                tunnel: w369 -> [w377 w380]
                frame "tif", "tiff" {
                  n166 = call "TIFFStream Write.vi"("File data"=w379, "Last image in file?"=TRUE, "Current and next IFD offset in"=w375, "Image data reference"=w377) -> ()  [unwired: 5 in, 3 out]
                }
                frame "bin", Default {
                  n167 = in-place {
                    in-place-border: w382 -> [w384]
                    in-place-border: [w383] -> w381
                    n168 = in-place-dvr #3(w380) -> (w386:u16[][])  [unwired: 1 out]
                    n169 = Write to Binary File(file (use dialog)=w384, data=w386, 5:FALSE ("prepend array or string size? (T)"), 9:T7."little-endian" ("byte order (0:big-endian, network order)")) -> (refnum out=w383:refnum<file>)  [unwired: 2 in, 2 out]
                    n170 = in-place-dvr #3(w386) -> ()  [unwired: 2 out]
                  }
                }
              }
            }
            frame True {
            }
          }
          n171 = case shown="False" w320 {
            tunnel: w319 -> [w364 _]
            tunnel: w315 -> [w363 _]
            tunnel: w317 -> [w362 _]
            tunnel: w318 -> [w361 _]
            frame False {
              n172 = case shown="\"tif\", \"tiff\"" w362 {
                tunnel: w364 -> [_ w368]
                tunnel: w363 -> [w366 w367]
                tunnel: w361 -> [w365 _]
                frame "tif", "tiff" {
                  n173 = call "TIFFStream Close.vi"("Image data reference"=w366, "File data"=w365) -> ()  [unwired: 9 in, 1 out]
                }
                frame "bin", Default {
                  n174 = Close File(refnum=w368) -> ()  [unwired: 1 in, 2 out]
                  n175 = Delete Data Value Reference(data value reference=w367) -> ()  [unwired: 1 in, 2 out]
                }
              }
            }
            frame True {
            }
          }
        }
        frame 1, Default {
          w479 = u16 0 items=["Stop", "Run"] ("RecordingState")
          w480 = u16 1 items=["Stop", "Run"] ("RecordingState")
          w486 = u32 0
          n176 = call <userlib>:"GetDescription.vi"("ph"=w495) -> ("ErrorOut"=w464:errorcluster, "Description"=w494:T10, "hout"=w466:u64)  [unwired: 3 in, 1 out]
          n177 = call <userlib>:"GetSizes.vi"("ph"=w466, "ErrorIn"=w464) -> ("hout"=w465:u64, "XResAct"=w459:u16, "YResAct"=w458:u16, "ErrorOut"=w463:errorcluster)  [unwired: 11 in, 3 out]
          n178 = Unbundle By Name(w494) -> ("DynResDESC"=w487:u16)
          n179 = To Long Integer(number=w459) -> (32bit integer=w469:i32)
          n180 = To Long Integer(number=w458) -> (32bit integer=w468:i32)
          n181 = call <userlib>:"SetRecordingState.vi"("ErrorIn"=w463, "RecordingState"=w480, "ph"=w465) -> ("ErrorOut"=w481:errorcluster, "hout"=w482:u64)  [unwired: 2 in, 1 out]
          n182 = Multiply(x=w469, y=w468) -> (x*y=w467:i32)
          n183 = call <userlib>:"AddBufferEX.vi"("ph"=w482, "BuffNr"=w483, "1stImage"=w486, "LastImage"=w486, "error in (no error)"=w481, "XRes"=w459, "YRes"=w458, "BitPerPixel"=w487) -> ("hout"=w490:u64, "error out"=w489:errorcluster)  [unwired: 5 in, 1 out]
          n184 = To Long Integer(number=w491) -> (32bit integer=w457:i32)
          n185 = call <vilib>:"Get File Extension.vi"("file"=w462) -> ("lowercase file extension"=w461:string)  [unwired: 6 in, 4 out]
          n186 = Initialize Array(u16 0 ("Element Data"), w467) -> (w492:u16[])
          n187 = Empty String/Path?(string/path=w462) -> (empty?=w471:bool)
          n188 = Not A Number/Path/Refnum?(number/path/refnum=w462) -> (NaN/Path/Refnum?=w472:bool)
          n189 = call <userlib>:"AddBufferEX.vi"("ph"=w490, "BuffNr"=w485, "1stImage"=w486, "LastImage"=w486, "error in (no error)"=w489, "XRes"=w459, "YRes"=w458, "BitPerPixel"=w487) -> ("hout"=w484:u64, "error out"=w488:errorcluster)  [unwired: 5 in, 1 out]
          n190 = Or(x=w471, y=w472) -> (x .or. y?=w470:bool)
          n191 = case shown="False" w470 {
            tunnel: w462 -> [w514 _]
            tunnel: [w513 refnum<file> refnum ("refnum out")] -> w474
            tunnel: w461 -> [w512 _]
            tunnel: [w511 _] -> w449
            tunnel: [w510 w537] -> w460
            tunnel: [w509 _] -> w453
            tunnel: w459 -> [w508 w540]
            tunnel: w458 -> [w507 w541]
            frame False {
              n192 = case shown="\"tif\", \"tiff\"" w512 {
                tunnel: w514 -> [w523 w534]
                tunnel: [refnum<file> refnum ("refnum out") w532] -> w513
                tunnel: [w522 _] -> w511
                tunnel: [w521 w527] -> w510
                tunnel: [w520 _] -> w509
                tunnel: w508 -> [w519 w525]
                tunnel: w507 -> [w518 w526]
                frame "tif", "tiff" {
                  n193 = To Unsigned Long Integer(number=w519) -> (unsigned 32bit integer=w516:u32)
                  n194 = To Unsigned Long Integer(number=w518) -> (unsigned 32bit integer=w517:u32)
                  n195 = call "TIFFStream Open.vi"("File path"=w523, "Height Pixels"=w517, "Width Pixels"=w516, "Big endian?"=FALSE) -> ("Current and next IFD offset"=w520:u32[], "Image data reference"=w521:refnum<data-value>, "File data"=w522:T11)  [unwired: 4 in, 1 out]
                }
                frame "bin", Default {
                  n196 = To Long Integer(number=w526) -> (32bit integer=w528:i32)
                  n197 = To Long Integer(number=w525) -> (32bit integer=w529:i32)
                  n198 = Open/Create/Replace File(file path (use dialog)=w534, operation (0:open)=T8."replace or create") -> (refnum out=w532:refnum<file>)  [unwired: 4 in, 2 out]
                  n199 = Initialize Array(u16 0 ("element"), w528, w529) -> (w530:u16[][])
                  n200 = New Data Value Reference(data value=w530) -> (data value reference=w527:refnum<data-value>)  [unwired: 1 in, 1 out]
                }
              }
            }
            frame True {
              n201 = To Long Integer(number=w541) -> (32bit integer=w535:i32)
              n202 = To Long Integer(number=w540) -> (32bit integer=w536:i32)
              n203 = Initialize Array(u16 0 ("element"), w535, w536) -> (w538:u16[][])
              n204 = New Data Value Reference(data value=w538) -> (data value reference=w537:refnum<data-value>)  [unwired: 1 in, 1 out]
            }
          }
          n205 = for {
            N: w457 -> [w557]
            tunnel: w484 -> [w579]
            tunnel: w493 -> [w577]
            tunnel: w462 -> [w575]
            tunnel: w492 -> [w574]
            tunnel: w483 -> [w571]
            tunnel: w487 -> [w570]
            tunnel: w458 -> [w564]
            tunnel: w459 -> [w565]
            tunnel: w485 -> [w566]
            tunnel: [w563] -> w476
            shift-right: [w561] -> w475
            shift-left: w488 -> [w580]
            tunnel: w474 -> [w560]
            tunnel: [w559] -> w473
            tunnel: w470 -> [w558]
            tunnel: w461 -> [w552]
            tunnel: w460 -> [w551]
            tunnel: [w553] -> w456
            tunnel: [w552] -> w455
            tunnel: w454 -> [w550]
            shift-right: [w548] -> w452
            shift-left: w453 -> [w549]
            tunnel: w451 -> [w547]
            border: w449 -> [_]
            tunnel: [w543] -> w450
            i -> [w556]
            stop <- w545 stop-if-true
            w567 = u32 0
            n206 = Not A Number/Path/Refnum?(number/path/refnum=w577) -> (NaN/Path/Refnum?=w578:bool)
            n207 = call <userlib>:"WaitForBuffer.vi"("ph"=w579, "sBufNr"=w571, "sBufNr 2"=w566, "timeout"=u32 3000, "error in (no error)"=w580) -> ("hout"=w582:u64, "Buffer_Ready"=w573:bool, "error out"=w572:errorcluster)  [unwired: 10 in, 2 out]
            n208 = Select(t=w571, s=w573, f=w566) -> (s? t:f=w569:i16)
            n209 = call <userlib>:"GetImageBuffer.vi"("ph"=w582, "BuffIn"=w574, "BuffNr"=w569, "error in (no error)"=w572, "xRes"=w565, "yRes"=w564, "Bitresolution"=w570) -> ("hout"=w568:u64, "BuffOut"=w583:u16[], "error out"=w562:errorcluster)  [unwired: 5 in, 1 out]
            n210 = in-place {
              in-place-border: w583 -> [w587]
              in-place-border: [w584] -> w576
              in-place-border: w565 -> [w586]
              in-place-border: w564 -> [w585]
              n211 = in-place-dvr #4(w551) -> ()  [unwired: 2 out]
              n212 = Reshape Array(w587, w585, w586) -> (w584:u16[][])
              n213 = in-place-dvr #4(w584) -> (w553:refnum<data-value>)  [unwired: 1 out]
            }
            n214 = case shown="False" w578 {
              tunnel: w577 -> [w621 _]
              tunnel: w553 -> [w620 _]
              tunnel: w550 -> [w619 _]
              frame False {
                n215 = in-place {
                  in-place-border: w621 -> [w624]
                  in-place-border: [w622] -> w618
                  n216 = in-place-dvr #5(w620) -> (w623:u16[][])  [unwired: 1 out]
                  n217 = call "IMAQ ArrayToImage"("Image Pixels (U16)"=w623, "Image"=w624) -> ("Image Out"=w622:T5)  [unwired: 8 in, 1 out]
                  n218 = in-place-dvr #5(w623) -> ()  [unwired: 2 out]
                }
                n219 = property class="ImageControl"(reference=w619, "Value"=w618) -> ()  [unwired: 1 in, 2 out]
              }
              frame True {
              }
            }
            n220 = call <userlib>:"AddBufferEX.vi"("ph"=w568, "BuffNr"=w569, "1stImage"=w567, "LastImage"=w567, "error in (no error)"=w562, "XRes"=w565, "YRes"=w564, "BitPerPixel"=w570) -> ("hout"=w563:u64, "error out"=w561:errorcluster)  [unwired: 5 in, 1 out]
            n221 = Decrement(x=w557) -> (x-1=w555:i32)
            n222 = property class="Bool (strict)"(reference=w547) -> ("Value"=w546:bool)  [unwired: 1 in, 2 out]
            n223 = Equal?(x=w555, y=w556) -> (x = y?=w554:bool)
            n224 = Not(x=w546) -> (.not. x?=w545:bool)
            n225 = feedback #6() -> (w543:T11)
            n226 = case shown="False" w558 {
              tunnel: w575 -> [_ _]
              tunnel: w576 -> [w597 _]
              tunnel: w560 -> [w596 w617]
              tunnel: [w595 w617] -> w559
              tunnel: w552 -> [w594 _]
              tunnel: w553 -> [w593 _]
              tunnel: w554 -> [w592 _]
              tunnel: w549 -> [w591 w616]
              tunnel: [w590 w616] -> w548
              tunnel: [w589 w615] -> w544
              tunnel: w543 -> [w588 w615]
              frame False {
                n227 = case shown="\"tif\", \"tiff\"" w594 {
                  tunnel: w597 -> [_ _]
                  tunnel: w596 -> [w604 w609]
                  tunnel: [w604 w608] -> w595
                  tunnel: w593 -> [w603 w607]
                  tunnel: w592 -> [w602 _]
                  tunnel: w591 -> [w601 w606]
                  tunnel: [w600 w606] -> w590
                  tunnel: [w599 w605] -> w589
                  tunnel: w588 -> [w598 w605]
                  frame "tif", "tiff" {
                    n228 = call "TIFFStream Write.vi"("File data"=w598, "Last image in file?"=w602, "Current and next IFD offset in"=w601, "Image data reference"=w603) -> ("Current and next IFD offset out"=w600:u32[], "File data out"=w599:T11)  [unwired: 5 in, 1 out]
                  }
                  frame "bin", Default {
                    n229 = in-place {
                      in-place-border: w609 -> [w611]
                      in-place-border: [w610] -> w608
                      n230 = in-place-dvr #7(w607) -> (w613:u16[][])  [unwired: 1 out]
                      n231 = Write to Binary File(file (use dialog)=w611, data=w613, 5:FALSE ("prepend array or string size? (T)"), 9:T7."little-endian" ("byte order (0:big-endian, network order)")) -> (refnum out=w610:refnum<file>)  [unwired: 2 in, 2 out]
                      n232 = in-place-dvr #7(w613) -> ()  [unwired: 2 out]
                    }
                  }
                }
              }
              frame True {
              }
            }
            n233 = feedback-in #6(w544) -> ()
          }
          n234 = case shown="False" w470 {
            tunnel: w473 -> [w501 _]
            tunnel: w456 -> [w500 _]
            tunnel: w455 -> [w499 _]
            tunnel: w450 -> [w498 _]
            tunnel: w452 -> [w497 _]
            frame False {
              n235 = case shown="\"False\"" w499 {
                tunnel: w501 -> [_ w506]
                tunnel: w500 -> [w504 w505]
                tunnel: w498 -> [w503 _]
                tunnel: w497 -> [w502 _]
                frame "False" {
                  n236 = call "TIFFStream Close.vi"("Current and next IFD offset"=w502, "Image data reference"=w504, "File data"=w503) -> ()  [unwired: 8 in, 1 out]
                }
                frame "bin", Default {
                  n237 = Close File(refnum=w506) -> ()  [unwired: 1 in, 2 out]
                  n238 = Delete Data Value Reference(data value reference=w505) -> ()  [unwired: 1 in, 2 out]
                }
              }
            }
            frame True {
            }
          }
          n239 = call <userlib>:"CancelImages.vi"("error in (no error)"=w475, "ph"=w476) -> ("error out"=w478:errorcluster, "hout"=w477:u64)  [unwired: 1 in, 1 out]
          n240 = call <userlib>:"SetRecordingState.vi"("ErrorIn"=w478, "RecordingState"=w479, "ph"=w477) -> ()  [unwired: 2 in, 3 out]
        }
      }
      n241 = To Variant(anything=w303) -> (Variant=w302:variant)
    }
    frame "Get status" {
      n242 = Bundle By Name(cluster=w631, "System OK?"=FALSE, "Temperature"=nan, "ROI"=cluster{"X":u32, "X2":u32, "Y":u32, "Y2":u32} {"X"=0, "X2"=1, "Y"=0, "Y2"=1}, "Binning"=cluster{"X":u32, "Y":u32} {"X"=1, "Y"=1}) -> (w630:T1)
    }
    frame "Other settings" {
      n243 = Variant To Data(type=w635, Variant=w639) -> (data=w634:T3)  [unwired: 1 in, 1 out]
      n244 = Unbundle By Name(w634) -> ("Handle"=w638:u64, "Buffers"=w632:i16[])
      n245 = call "PCO Edge_Settings.vi"("Buffers"=w632, "Handle"=w638) -> ("Handle Out"=w636:u64)  [unwired: 9 in]
      n246 = Bundle By Name(cluster=w634, "Handle"=w636) -> (w637:T3)
      n247 = To Variant(anything=w637) -> (Variant=w633:variant)
    }
  }
  "Status" <- w8
  "Camera-specific out" <- w3
